vi "(SubVI)GPIO Trigger Picture.vi"(7 "num of ch (4)":i32=4, 8 "pulse height (24)":i16=24, 9 "vertical interval (6)":i16=6, 10 "box width (120)":i16=120, 11 "Trig Ctrl":T1={"1st Trig"={"Trigger"=TRUE, "Low"=0, "High"=100}, "2nd Trig"={"Trigger"=TRUE, "Low"=0, "High"=100}, "3rd Trig"={"Trigger"=TRUE, "Low"=0, "High"=100}, "4th Trig"={"Trigger"=TRUE, "Low"=0, "High"=100}} {"4th Trig"."High" min=1 max=8000; "4th Trig"."Low" max=7999; "3rd Trig"."High" min=1 max=8000; "3rd Trig"."Low" max=7999; "2nd Trig"."High" min=1 max=8000; "2nd Trig"."Low" max=7999; "1st Trig"."High" min=1 max=8000; "1st Trig"."Low" max=7999}) -> (3 "picture":picture)   [LabVIEW 2020]
uses:
  System Command/Controls/(Ctrl)System Command_Trig GPIO Control.ctl
panel:
  # "L1"
  # "H1"
  # "L2"
  # "H2"
  # "L3"
  # "H3"
  # "Trigger"
  # "L (us)"
  # "H (us)"
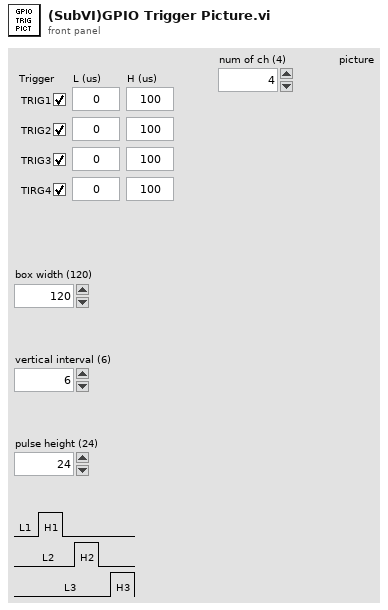
[diagram p1: front panel]
types:
  T1 = typedef "(Ctrl)System Command_Trig GPIO Control.ctl" = cluster{"1st Trig":cluster{"Trigger":bool, "Low":u16, "High":u16}, "2nd Trig":cluster{"Trigger":bool, "Low":u16, "High":u16}, "3rd Trig":cluster{"Trigger":bool, "Low":u16, "High":u16}, "4th Trig":cluster{"Trigger":bool, "Low":u16, "High":u16}}
  T2 = cluster{"horizontal":enum16{"left", "center", "right"}, "vertical":enum16{"top", "center", "bottom"}}
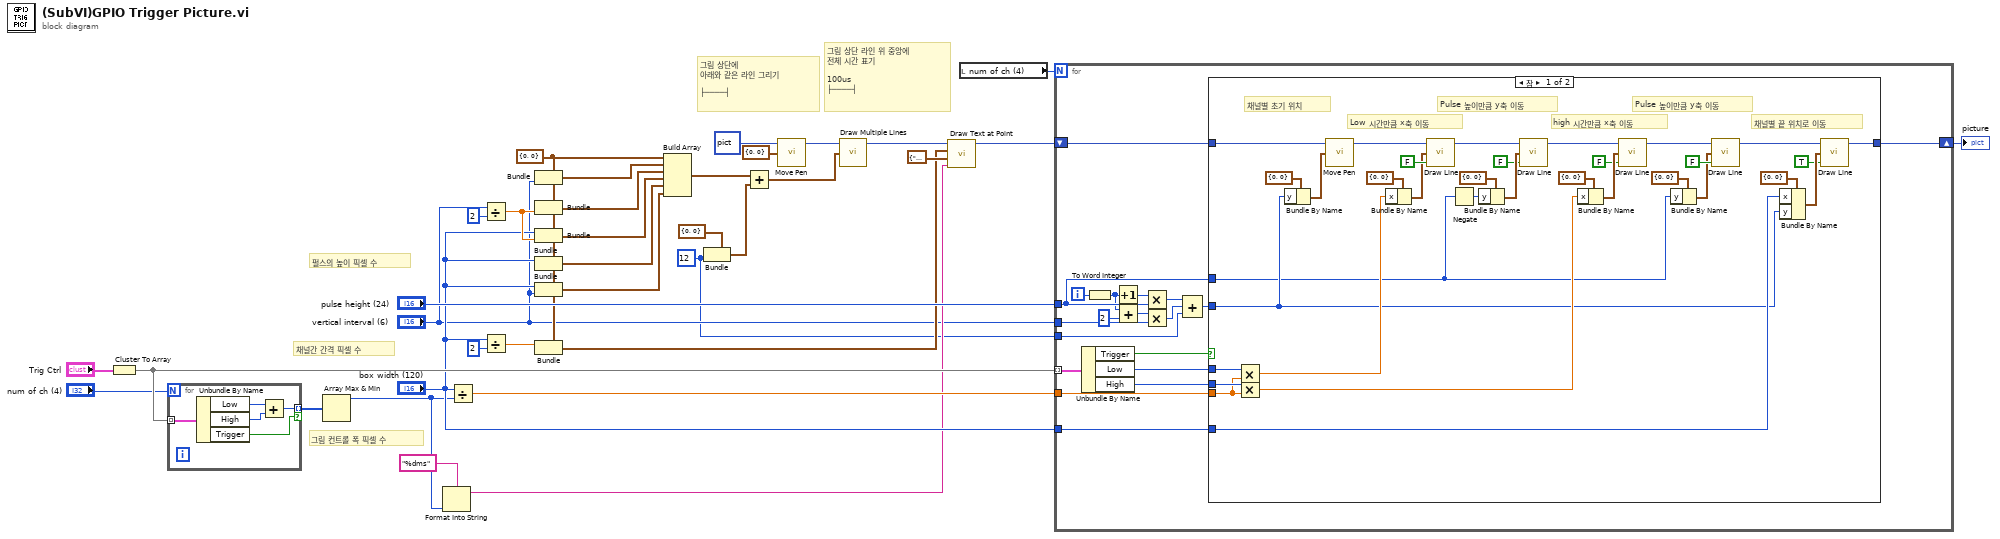
[diagram p0: block diagram]
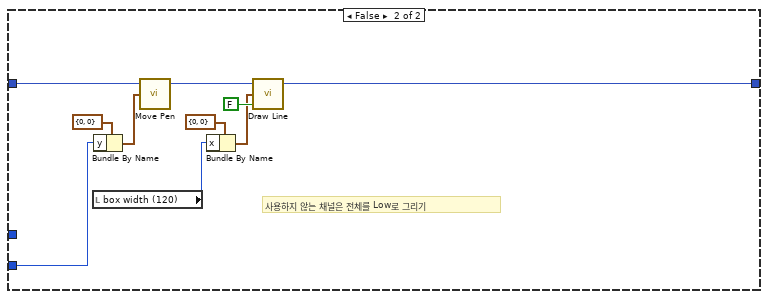
[diagram p2: hidden frame]
diagram:
  w3 = i16 12 ("y")
  w13 = cluster{"x":i16, "y":i16} {"x"=0, "y"=0} ("new position")
  # "그림 상단에 \n아래와 같은 라인 그리기\n\n├────┤"
  # "그림 상단 라인 위 중앙에\n전체 시간 표기\n\n100us\n├────┤"
  # "그림 컨트롤 폭 픽셀 수"
  # "채널간 간격 픽셀 수"
  # "펄스의 높이 픽셀 수"
  n1 = Cluster To Array(cluster="Trig Ctrl") -> (array=w34:cluster{"Trigger":bool, "Low":u16, "High":u16}[])
  n2 = for {
    N: "num of ch (4)" -> [_]
    tunnel: w34 -> [w40] mode=indexing
    tunnel: [w37] -> w33 mode=indexing if=w36
    n3 = Unbundle By Name(w40) -> ("Low"=w39:u16, "High"=w38:u16, "Trigger"=w36:bool)
    n4 = Add(x=w39, y=w38) -> (x+y=w37:u16)
  }
  n5 = Array Max & Min(array=w33) -> (max value=w11:u16)  [unwired: 3 out]
  n6 = Format Into String(format string="%dms" ("포맷 문자열"), w11) -> (resulting string=w9:string)  [unwired: 2 in, 1 out]
  n7 = Divide(x="box width (120)", y=w11) -> (x/y=w31:dbl)
  n8 = Divide(x="vertical interval (6)", y=i16 2) -> (x/y=w25:dbl)
  n9 = Divide(x="box width (120)", y=i16 2) -> (x/y=w8:dbl)
  n10 = Bundle(cluster=w13, "y"="vertical interval (6)") -> (w24:cluster{"x":i16, "y":i16})  [unwired: 1 in]
  n11 = Bundle(cluster=w13, "y"=w25) -> (w23:cluster{"x":i16, "y":i16})  [unwired: 1 in]
  n12 = Bundle(cluster=w13, "x"="box width (120)", "y"=w25) -> (w22:cluster{"x":i16, "y":i16})
  n13 = Bundle(cluster=w13, "x"="box width (120)") -> (w21:cluster{"x":i16, "y":i16})  [unwired: 1 in]
  n14 = Bundle(cluster=w13, "x"="box width (120)", "y"="vertical interval (6)") -> (w20:cluster{"x":i16, "y":i16})
  n15 = Bundle(cluster=w13, "x"=w8) -> (w12:cluster{"x":i16, "y":i16})  [unwired: 1 in]
  n16 = Build Array(w13, w24, w23, w22, w21, w20) -> (w19:cluster{"x":i16, "y":i16}[])
  n17 = Bundle(cluster=cluster{"x":i16, "y":i16} {"x"=0, "y"=0} ("new position"), "y"=w3) -> (w4:cluster{"x":i16, "y":i16})  [unwired: 1 in]
  n18 = Add(x=w19, y=w4) -> (x+y=w7:cluster{"x":i16, "y":i16}[])
  n19 = call <vilib>:"Move Pen.vi"("new position"=cluster{"x":i16, "y":i16} {"x"=0, "y"=0}, "picture"=picture data[5B]) -> ("new picture"=w27:picture)  [unwired: 3 in]
  n20 = call <vilib>:"Draw Multiple Lines.vi"("picture"=w27, "line endpoints"=w7) -> ("new picture"=w18:picture)  [unwired: 7 in]
  n21 = call <vilib>:"Draw Text at Point.vi"("text"=w9, "alignment(left, top)"=T2 {"horizontal"=enum."center", "vertical"=enum."top"}, "origin"=w12, "picture"=w18) -> ("new picture"=w17:picture)  [unwired: 6 in, 1 out]
  n22 = local read "num of ch (4)"() -> (w2:i32)
  n23 = for {
    N: w2 -> [_]
    tunnel: w34 -> [w59] mode=indexing
    shift-right: [w54] -> w30
    shift-left: w17 -> [w55]
    tunnel: "vertical interval (6)" -> [w52]
    tunnel: "pulse height (24)" -> [w48]
    tunnel: w31 -> [w47]
    tunnel: "box width (120)" -> [w46]
    tunnel: w3 -> [w41]
    i -> [w53]
    n24 = Unbundle By Name(w59) -> ("Trigger"=w58:bool, "Low"=w57:u16, "High"=w56:u16)
    n25 = To Word Integer(number=w53) -> (16bit integer=w44:i16)
    n26 = Increment(x=w44) -> (x+1=w45:i16)
    n27 = Add(x=w44, y=i16 2) -> (x+y=w42:i16)
    n28 = Multiply(x=w45, y=w48) -> (x*y=w51:i16)
    n29 = Multiply(x=w42, y=w52) -> (x*y=w50:i16)
    n30 = Compound Arithmetic op=ADD(w51, w50, w41) -> (w49:i16)
    n31 = case shown="참" w58 {
      tunnel: w57 -> [w88 _]
      tunnel: w56 -> [w79 _]
      tunnel: w49 -> [w62 w95]
      tunnel: w55 -> [w92 w102]
      tunnel: [w65 w94] -> w54
      tunnel: w48 -> [w60 _]
      tunnel: w47 -> [w78 _]
      tunnel: w46 -> [w63 _]
      frame True {
        # "채널별 끝 위치로 이동"
        # "Pulse 높이만큼 y축 이동"
        # "high 시간만큼 x축 이동"
        # "Pulse 높이만큼 y축 이동"
        # "Low 시간만큼 x축 이동"
        # "채널별 초기 위치"
        n32 = Multiply(x=w88, y=w78) -> (x*y=w85:dbl)
        n33 = Multiply(x=w79, y=w78) -> (x*y=w69:dbl)
        n34 = Bundle By Name(cluster=cluster{"x":i16, "y":i16} {"x"=0, "y"=0} ("new position"), "y"=w62) -> (w89:cluster{"x":i16, "y":i16})
        n35 = call <vilib>:"Move Pen.vi"("new position"=w89, "picture"=w92) -> ("new picture"=w91:picture)  [unwired: 3 in]
        n36 = Bundle By Name(cluster=cluster{"x":i16, "y":i16} {"x"=0, "y"=0} ("new position"), "x"=w85) -> (w84:cluster{"x":i16, "y":i16})
        n37 = call <vilib>:"Draw Line.vi"("picture"=w91, "end point"=w84, "absolute coordinates?(T)"=FALSE) -> ("new picture"=w80:picture)  [unwired: 6 in]
        n38 = Negate(x=w60) -> (-x=w61:i16)
        n39 = Bundle By Name(cluster=cluster{"x":i16, "y":i16} {"x"=0, "y"=0} ("new position"), "y"=w61) -> (w83:cluster{"x":i16, "y":i16})
        n40 = call <vilib>:"Draw Line.vi"("picture"=w80, "end point"=w83, "absolute coordinates?(T)"=FALSE) -> ("new picture"=w70:picture)  [unwired: 6 in]
        n41 = Bundle By Name(cluster=cluster{"x":i16, "y":i16} {"x"=0, "y"=0} ("new position"), "x"=w69) -> (w73:cluster{"x":i16, "y":i16})
        n42 = call <vilib>:"Draw Line.vi"("picture"=w70, "end point"=w73, "absolute coordinates?(T)"=FALSE) -> ("new picture"=w77:picture)  [unwired: 6 in]
        n43 = Bundle By Name(cluster=cluster{"x":i16, "y":i16} {"x"=0, "y"=0} ("new position"), "y"=w60) -> (w74:cluster{"x":i16, "y":i16})
        n44 = call <vilib>:"Draw Line.vi"("picture"=w77, "end point"=w74, "absolute coordinates?(T)"=FALSE) -> ("new picture"=w64:picture)  [unwired: 6 in]
        n45 = Bundle By Name(cluster=cluster{"x":i16, "y":i16} {"x"=0, "y"=0} ("new position"), "x"=w63, "y"=w62) -> (w68:cluster{"x":i16, "y":i16})
        n46 = call <vilib>:"Draw Line.vi"("picture"=w64, "end point"=w68, "absolute coordinates?(T)"=TRUE) -> ("new picture"=w65:picture)  [unwired: 6 in]
      }
      frame False {
        # "사용하지 않는 채널은 전체를 Low로 그리기"
        n47 = local read "box width (120)"() -> (w93:i16)
        n48 = Bundle By Name(cluster=cluster{"x":i16, "y":i16} {"x"=0, "y"=0} ("new position"), "y"=w95) -> (w99:cluster{"x":i16, "y":i16})
        n49 = call <vilib>:"Move Pen.vi"("new position"=w99, "picture"=w102) -> ("new picture"=w101:picture)  [unwired: 3 in]
        n50 = Bundle By Name(cluster=cluster{"x":i16, "y":i16} {"x"=0, "y"=0} ("new position"), "x"=w93) -> (w96:cluster{"x":i16, "y":i16})
        n51 = call <vilib>:"Draw Line.vi"("picture"=w101, "end point"=w96, "absolute coordinates?(T)"=FALSE) -> ("new picture"=w94:picture)  [unwired: 6 in]
      }
    }
  }
  "picture" <- w30
